vi "Check Sensors.vi"(8 "error in (no error)":errorcluster, 11 "App Data in":T1={"Pump Station Controls"={"Lag Pump"=enum."OFF", "Lead Pump"=enum."OFF", "ALARM"=0.0, "LAG"=0.0, "LEAD"=0.0, "STOP"=0.0}, "Pump Indicators"={"Pump Water Level"=0.0, "ALARM"=FALSE, "LAG"=FALSE, "LEAD"=FALSE, "STOP"=FALSE, "PUMP 1 STATE"=FALSE, "PUMP 2 STATE"=FALSE}, "Alarm"=refnum, "Lag Start Time"=timestamp(0 s since 1904-01-01), "Lead Start Time"=timestamp(0 s since 1904-01-01), "Main Q"=refnum} {"Pump Indicators"."Pump Water Level" scale=0.0..4.0}) -> (0 "error out":errorcluster, 3 "App Data in 2":T1={"Pump Station Controls"={"Lag Pump"=enum."OFF", "Lead Pump"=enum."OFF", "ALARM"=0.0, "LAG"=0.0, "LEAD"=0.0, "STOP"=0.0}, "Pump Indicators"={"Pump Water Level"=0.0, "ALARM"=FALSE, "LAG"=FALSE, "LEAD"=FALSE, "STOP"=FALSE, "PUMP 1 STATE"=FALSE, "PUMP 2 STATE"=FALSE}, "Alarm"=refnum, "Lag Start Time"=timestamp(0 s since 1904-01-01), "Lead Start Time"=timestamp(0 s since 1904-01-01), "Main Q"=refnum} {"Pump Indicators"."Pump Water Level" scale=0.0..4.0})   [LabVIEW 2024]
uses:
  App Data.ctl
  Pump Controls.ctl
  Pump Switch.ctl
  Pump Indicators.ctl
  Q Info.ctl
  a115a477-68aa-4495-a681-da1562e3485a.vi
  201dc78a-b6da-45c8-aa32-36506b213544.vi
  a11d1513-fd79-4290-a36f-63a9e0f3eaad.vi
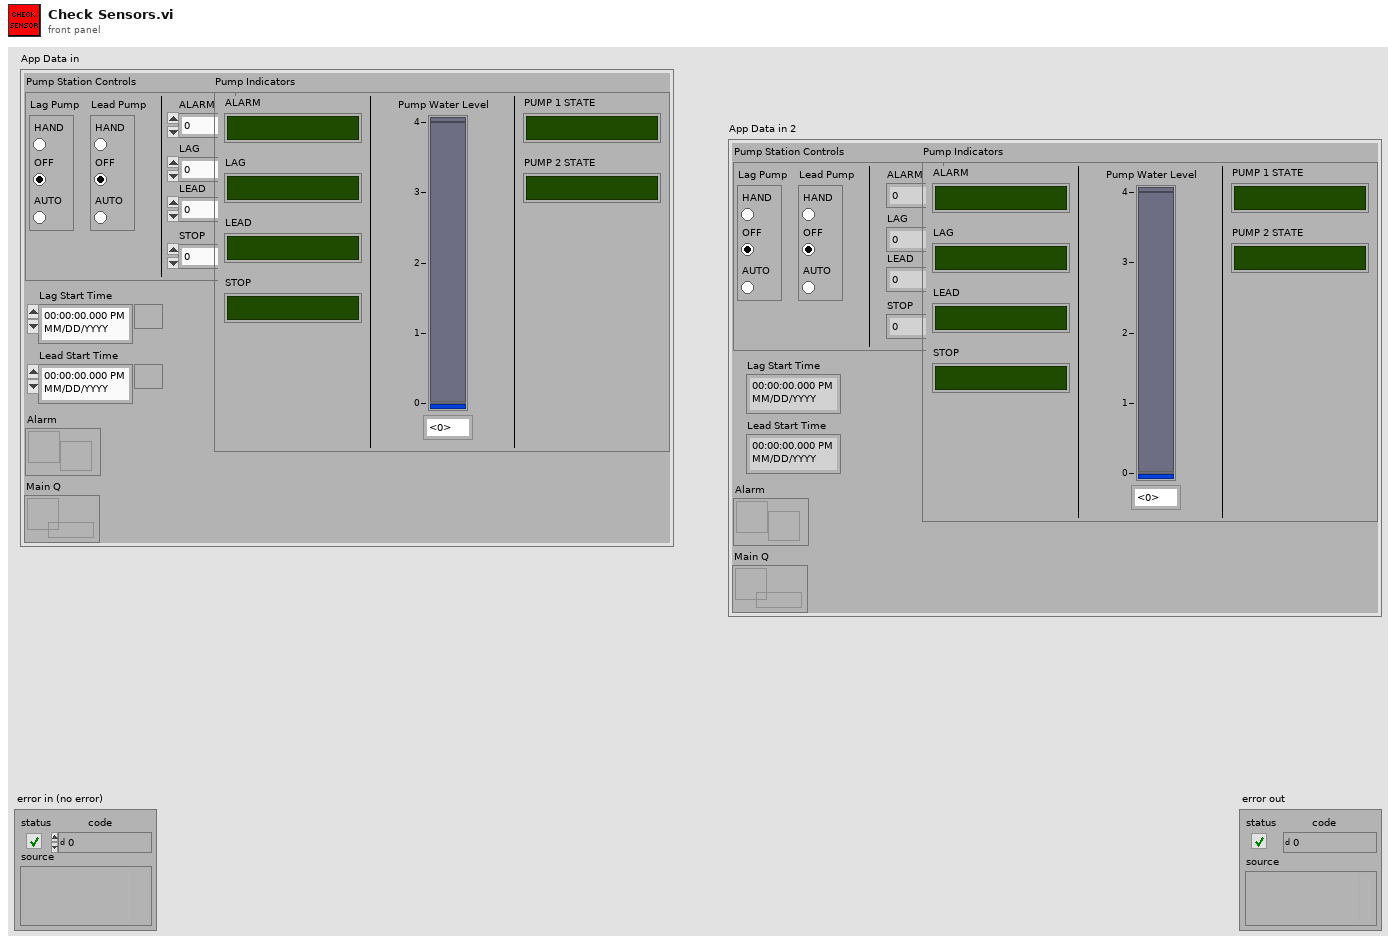
[diagram p1: front panel]
types:
  T1 = typedef "App Data.ctl" = cluster{"Pump Station Controls":T2, "Pump Indicators":T4, "Alarm":refnum<notifier>, "Lag Start Time":timestamp, "Lead Start Time":timestamp, "Main Q":refnum<queue>}
  T2 = typedef "Pump Controls.ctl" = cluster{"Lag Pump":T3, "Lead Pump":T3, "ALARM":dbl, "LAG":dbl, "LEAD":dbl, "STOP":dbl}
  T3 = typedef "Pump Switch.ctl" = enum32{"HAND", "OFF", "AUTO"}
  T4 = typedef "Pump Indicators.ctl" = cluster{"Pump Water Level":dbl, "ALARM":bool, "LAG":bool, "LEAD":bool, "STOP":bool, "PUMP 1 STATE":bool, "PUMP 2 STATE":bool}
  T5 = typedef "Q Info.ctl" = cluster{"State":string, "Data":variant}
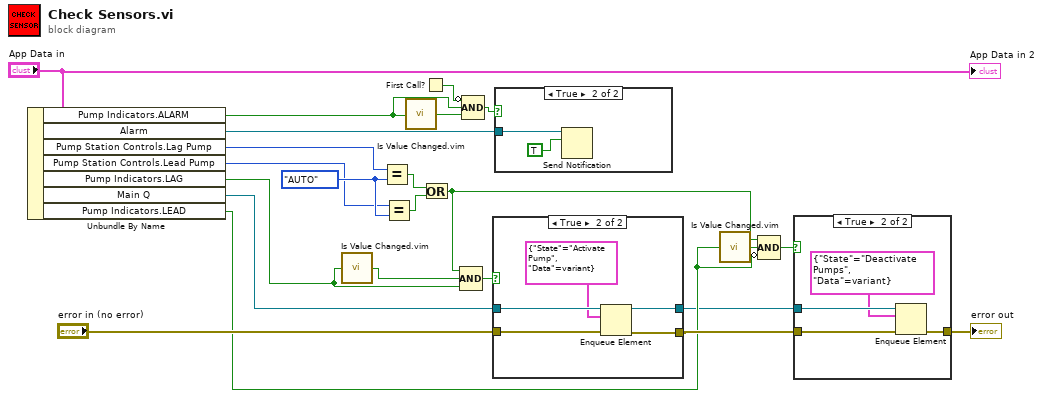
[diagram p0: block diagram]
diagram:
  w16 = Pump_Switch."AUTO" ("y")
  n1 = Unbundle By Name("App Data in") -> ("Pump Indicators.ALARM"=w19:bool, "Alarm"=w22:refnum<notifier>, "Pump Station Controls.Lag Pump"=w17:T3, "Pump Station Controls.Lead Pump"=w15:T3, "Pump Indicators.LAG"=w10:bool, "Main Q"=w11:refnum<queue>, "Pump Indicators.LEAD"=w3:bool)
  n2 = call "Is Value Changed.vim"("value"=w10) -> ("changed or first call?"=w9:bool)
  n3 = Equal?(x=w17, y=w16) -> (x = y?=w13:bool)
  n4 = Equal?(x=w15, y=w16) -> (x = y?=w14:bool)
  n5 = call "Is Value Changed.vim"("value"=w19) -> ("changed or first call?"=w20:bool)
  n6 = First Call?() -> (First Call?: T/F=w18:bool)
  n7 = Or(x=w13, y=w14) -> (x .or. y?=w2:bool)
  n8 = Compound Arithmetic op=AND(w2, w9, w10) -> (w8:bool)
  n9 = Compound Arithmetic op=AND(invert w18, w19, w20) -> (w21:bool)
  n10 = case shown="True" w8 {
    tunnel: "error in (no error)" -> [w25 w30]
    tunnel: w11 -> [w24 w29]
    tunnel: [w25 w27] -> w7
    tunnel: [w24 w26] -> w1
    frame False {
    }
    frame True {
      n11 = Enqueue Element(queue=w29, element=T5 {"State"="Activate Pump", "Data"=variant}, error in (no error)=w30) -> (queue out=w26:refnum<queue>, error out=w27:errorcluster)  [unwired: 1 in, 1 out]
    }
  }
  n12 = case shown="True" w21 {
    tunnel: w22 -> [_ w32]
    frame False {
    }
    frame True {
      n13 = Send Notification(notification=TRUE, notifier=w32) -> ()  [unwired: 1 in, 2 out]
    }
  }
  n14 = call "Is Value Changed.vim"("value"=w3) -> ("changed or first call?"=w4:bool)
  n15 = Compound Arithmetic op=AND(w2, w4, invert w3) -> (w5:bool)
  n16 = case shown="True" w5 {
    tunnel: w7 -> [w33 w36]
    tunnel: [w33 w37] -> w6
    tunnel: w1 -> [_ w35]
    frame False {
    }
    frame True {
      n17 = Enqueue Element(queue=w35, element=T5 {"State"="Deactivate Pumps", "Data"=variant}, error in (no error)=w36) -> (error out=w37:errorcluster)  [unwired: 1 in, 2 out]
    }
  }
  "error out" <- w6
  "App Data in 2" <- "App Data in"
